vi "Rename Subdiagram Label.vi"(7 "Evaluation String":string, 8 "error in (no error)":errorcluster, 11 "SubVI Reference":refnum<vi>) -> (0 "error out":errorcluster)   [LabVIEW 2018]
doc: "Finds the disable structure surrounding the assert vi and renames the subdiagram label in the correct case to the evaluation string"
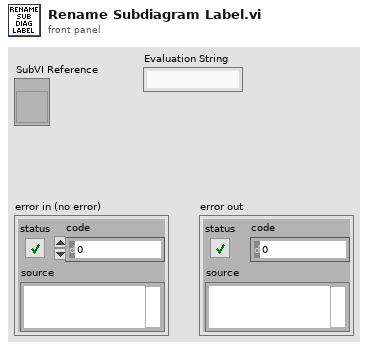
[diagram p1: front panel]
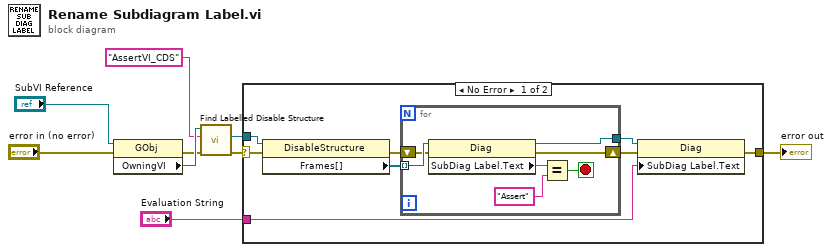
[diagram p0: block diagram]
diagram:
  n1 = property class="GObj"(reference="SubVI Reference", error in="error in (no error)") -> (error out=w7:errorcluster, "OwningVI"=w9:refnum<vi>)  [unwired: 1 out]
  n2 = call "Find Labelled Disable Structure.vi"("error in (no error)"=w7, "Label"="AssertVI_CDS", "VI in"=w9) -> ("error out"=w4:errorcluster, "DisableStructure Refnum"=w1:refnum<vi>)  [unwired: 6 in, 1 out]
  n3 = case shown="No Error" w4 {
    selector: w4 -> [w11 w25]
    tunnel: "Evaluation String" -> [w16 _]
    tunnel: [w12 w25] -> w6
    tunnel: w1 -> [w10 _]
    frame No Error {
      n4 = property class="DisableStructure"(reference=w10, error in=w11) -> (error out=w14:errorcluster, "Frames[]"=w13:refnum<vi>[])  [unwired: 1 out]
      n5 = for {
        tunnel: w13 -> [w24] mode=indexing
        tunnel: [w20] -> w17
        shift-right: [w19] -> w15
        shift-left: w14 -> [w18]
        stop <- w21 stop-if-true
        n6 = property class="Diag"(reference=w24, error in=w18) -> (reference out=w20:refnum<vi>, error out=w19:errorcluster, "SubDiag Label.Text"=w23:string)
        n7 = Equal?(x=w23, y="Assert") -> (x = y?=w21:bool)
      }
      n8 = property class="Diag"(reference=w17, error in=w15, "SubDiag Label.Text"=w16) -> (error out=w12:errorcluster)  [unwired: 1 out]
    }
    frame Error {
    }
  }
  "error out" <- w6
